vi "指数电流信号.vi"() -> ()   [LabVIEW 2020]
doc: "I. Description:\nThis example demonstrates how to acquire a continuous amount of data (Waveform) using the DAQ device's internal clock.\n\nII. Instructions for Running:\n1. Select the physical channel to correspond to where your signal is input on the DAQ device.\n2. Enter the minimum and maximum voltages.\nNote: For better accuracy try to match the input range to the expected voltage level of the measured signal.\n3. Select the number of samples to acquire per loop iteration.\n4. Set the rate of the acquisition\nNote: The rate should be AT LEAST twice as fast as the maximum frequency component of the signal being acquired.\n\nIII. Block Diagram Steps:\n1. Create an analog input voltage channel.\n2. Set the rate for the sample clock. Additionally, define the sample mode to be continuous.\n3. Call the Start VI to start the acquisition.\n4. Read the waveform data in a loop until the user hits the stop button or an error occurs.\nNote: This example reads data from one or more channels and returns an array of data. Use the Index Array function to access an individual channel of data.\n5. Call the Clear Task VI to clear the Task.\n6. Use the popup dialog box to display an error if any.\n\nIV. I/O Connections Overview:\nMake sure your signal input terminal matches the Physical Channel I/O Control. For further connection information, refer to your hardware reference manual."
uses:
  GlobalVariable.vi
  <vilib>/Analysis/polynomials.llb/Scalar Polynomial Evaluation (DBL).vi
  <vilib>/Analysis/NI_AALPro.lvlib
panel:
  out "实际步长(mS)":u32
  in  "定值电流观测":bool
  in  "二倍周期(秒)":dbl=80.0
  in  "开始自检":bool
  in  "初始I(0)电流(A)":dbl=1e-09
  in  "停止":bool
  in  "当前电流值（A)":dbl format="%#_6e"
  out "偏压(V)":dbl
  out "VI量程":bool[](array[boolean])
  in  "Loop Time (ms)":u32=200 caption="点间隔步长(mS)"
  out "XY Graph":cluster{"Y":dbl[], "Y":dbl[]}[](graph) caption="指数电流输出"
  # "I(t)=I(0)exp(t/Te)"
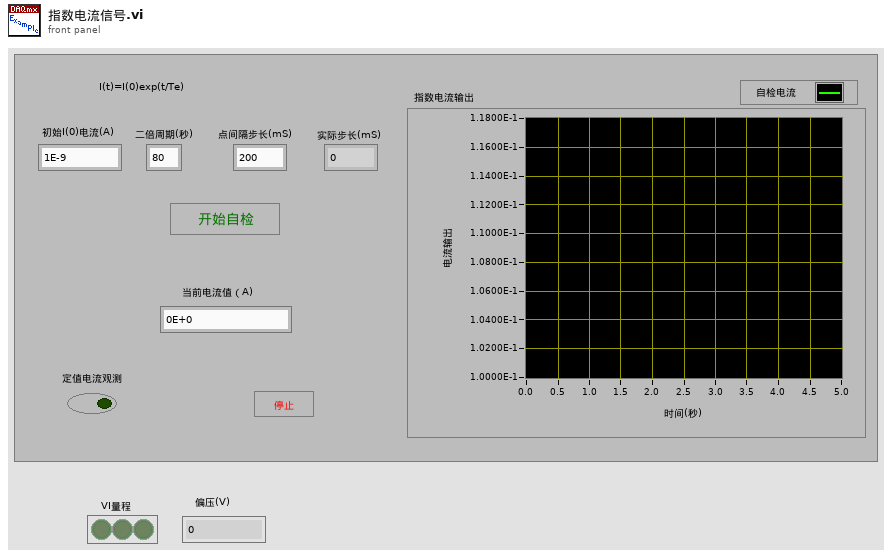
[diagram p1: front panel]
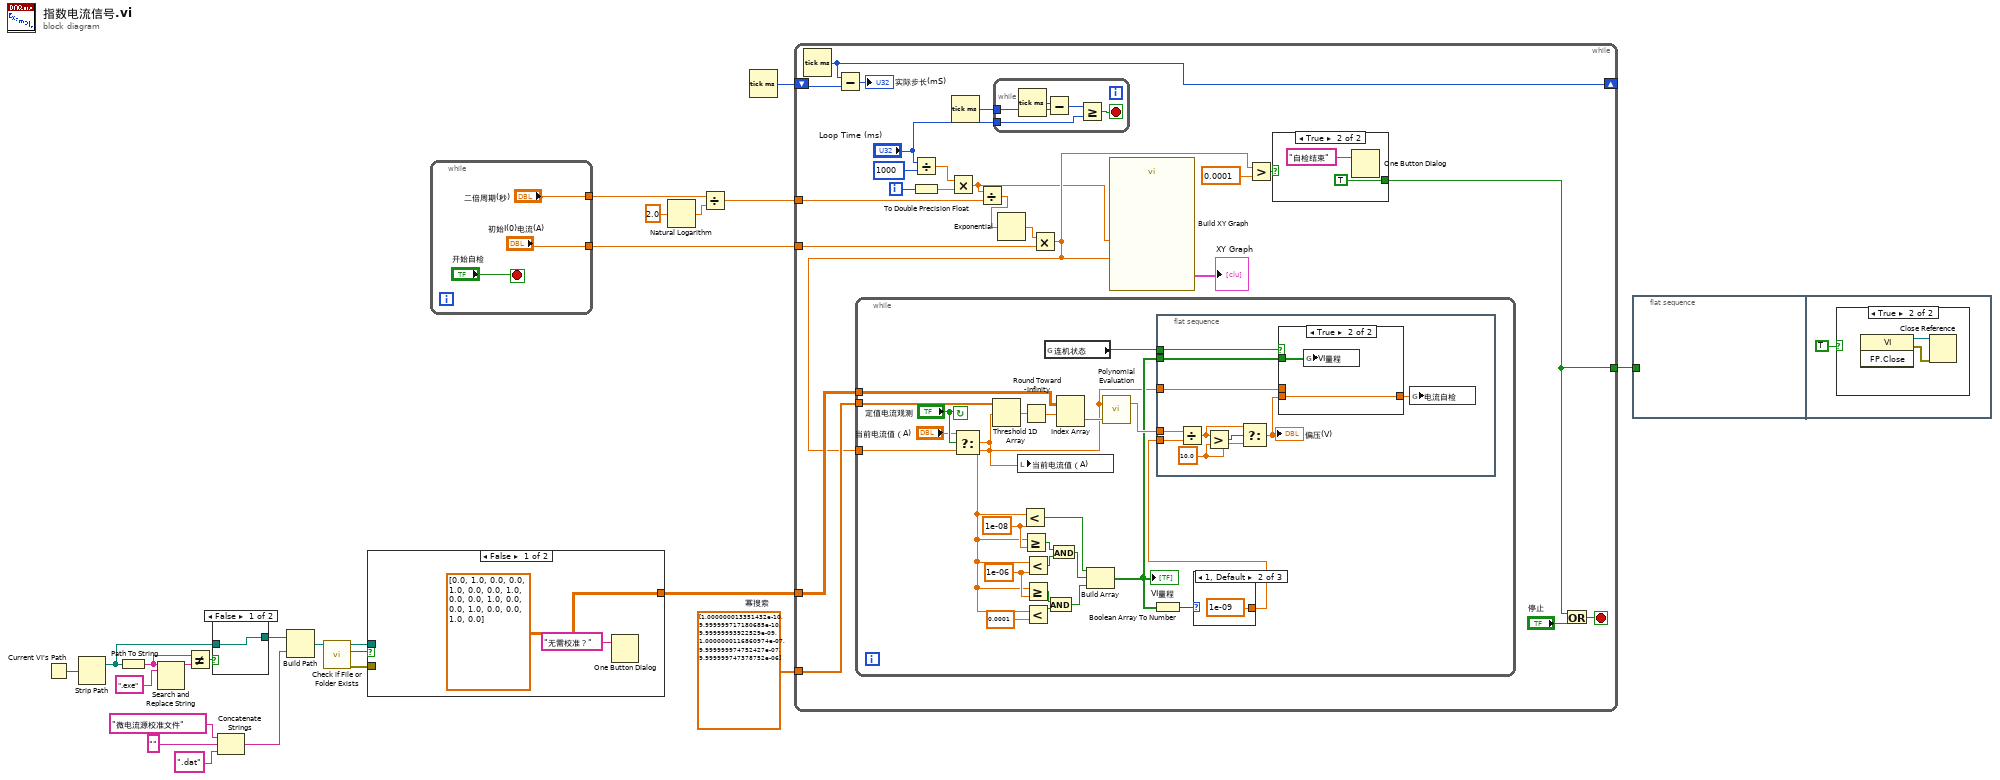
[diagram p0: block diagram]
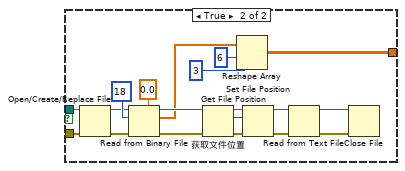
[diagram p2: hidden frame]
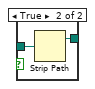
[diagram p4: hidden frame]
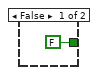
[diagram p5: hidden frame]
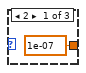
[diagram p7: hidden frame]
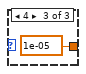
[diagram p8: hidden frame]
diagram:
  w20 = sgl[] [1e-10, 1e-09, 1e-08, 1e-07, 1e-06, 1e-05]  # 幂搜索
  n1 = Current VI's Path() -> (path=w19:path)
  n2 = Strip Path(path=w19) -> (stripped path=w14:path)  [unwired: 1 out]
  n3 = Path To String(path=w14) -> (string=w16:string)
  n4 = Search and Replace String(input string=w16, search string=".exe" ("搜索字符串")) -> (result string=w17:string)  [unwired: 6 in, 3 out]
  n5 = Not Equal?(x=w16, y=w17) -> (x != y?=w15:bool)
  n6 = case shown="False" w15 {
    tunnel: w14 -> [w25 w27]
    tunnel: [w25 w26] -> w13
    frame False {
    }
    frame True {
      n7 = Strip Path(path=w27) -> (stripped path=w26:path)  [unwired: 1 out]
    }
  }
  n8 = Concatenate Strings("微电流源校准文件", "" ("字符串"), ".dat") -> (w8:string)
  n9 = Build Path(base path=w13, name or relative path=w8) -> (appended path=w7:path)
  n10 = call <vilib>:"Check if File or Folder Exists.vi"("path"=w7) -> ("error out"=w4:errorcluster, "file or folder exists?"=w5:bool, "dup path"=w6:path)  [unwired: 8 in]
  n11 = case shown="False" w5 {
    tunnel: [sgl[][] [[0.0, 1.0, 0.0], [0.0, 1.0, 0.0], [0.0, 1.0, 0.0], [0.0, 1.0, 0.0], [0.0, 1.0, 0.0], [0.0, 1.0, 0.0]] w32] -> w12
    tunnel: w6 -> [_ w31]
    tunnel: w4 -> [_ w30]
    frame False {
      n12 = One Button Dialog(message="无需校准？" ("消息")) -> ()  [unwired: 1 in, 1 out]
    }
    frame True {
      n13 = Open/Create/Replace File(file path (use dialog)=w31, error in=w30) -> (refnum out=w37:refnum<file>, error out=w36:errorcluster)  [unwired: 4 in, 1 out]
      n14 = Read from Binary File(5:sgl 0.0 ("byte stream type"), 8:w36, 10:18 ("count"), 11:w37) -> (0:w39:errorcluster, 2:w35:sgl[], 3:w38:refnum<file>)  [unwired: 2 in, 1 out]
      n15 = Get File Position "获取文件位置"(4:w39, 7:w38) -> (0:w47:errorcluster, 2:w46:i64, 3:w48:refnum<file>)
      n16 = Reshape Array(w35, 6 ("维数大小"), 3 ("维数大小")) -> (w32:sgl[][])
      n17 = Set File Position(offset (in bytes) (0)=w46, refnum=w48, error in=w47) -> (refnum out=w45:refnum<file>, error out=w44:errorcluster)  [unwired: 1 in]
      n18 = Read from Text File(file (use dialog)=w45, error in=w44) -> (refnum out=w43:refnum<file>, error out=w42:errorcluster)  [unwired: 1 in, 3 out]
      n19 = Close File(refnum=w43, error in=w42) -> ()  [unwired: 2 out]
    }
  }
  n20 = while {
    tunnel: ["二倍周期(秒)"] -> w22
    tunnel: ["初始I(0)电流(A)"] -> w3
    stop <- "开始自检" stop-if-true
  }
  n21 = Natural Logarithm(1:2.0 ("x")) -> (0:w24:dbl)
  n22 = Divide(x=w22, y=w24) -> (x/y=w21:dbl)
  n23 = Tick Count (ms)() -> (millisecond timer value=w11:u32)
  n24 = while {
    tunnel: w21 -> [w66]
    tunnel: w3 -> [w65]
    tunnel: w12 -> [w63]
    tunnel: w20 -> [w62]
    shift-right: [w54] -> _
    shift-left: w11 -> [w58]
    tunnel: [w52] -> w1
    i -> [w64]
    stop <- w74 stop-if-true
    n25 = Tick Count (ms)() -> (millisecond timer value=w54:u32)
    n26 = Subtract(x=w54, y=w58) -> (x-y=→"实际步长(mS)":u32)
    n27 = Divide(x="Loop Time (ms)", y=u32 1000) -> (x/y=w68:dbl)
    n28 = To Double Precision Float(number=w64) -> (double precision float=w72:dbl)
    n29 = Multiply(x=w68, y=w72) -> (x*y=w55:dbl)
    n30 = Tick Count (ms)() -> (millisecond timer value=w56:u32)
    n31 = Divide(x=w55, y=w66) -> (x/y=w71:dbl)
    n32 = while {
      tunnel: w56 -> [w78]
      tunnel: "Loop Time (ms)" -> [w75]
      stop <- w76 stop-if-true
      n33 = Tick Count (ms)() -> (millisecond timer value=w79:u32)
      n34 = Subtract(x=w79, y=w78) -> (x-y=w77:u32)
      n35 = Greater Or Equal?(x=w77, y=w75) -> (x >= y?=w76:bool)
    }
    n36 = Exponential(1:w71) -> (0:w70:dbl)
    n37 = Multiply(x=w70, y=w65) -> (x*y=w61:dbl)
    n38 = while {
      tunnel: w61 -> [w93]
      tunnel: w63 -> [w89]
      tunnel: w62 -> [w91]
      stop <- "定值电流观测" continue-if-true
      w102 = 1e-06 ("y")
      w105 = 1e-08 ("y")
      n39 = Select(t="当前电流值（A)", s="定值电流观测", f=w93) -> (s? t:f=w84:dbl)
      n40 = Threshold 1D Array(2:w84, 3:w91) -> (0:w90:sgl)  [unwired: 1 in]
      n41 = local write "当前电流值（A)"(w84) -> ()
      n42 = Less?(x=w84, y=w105) -> (x < y?=w98:bool)
      n43 = Round Toward -Infinity(1:w90) -> (0:w88:sgl)
      n44 = Greater Or Equal?(x=w84, y=w105) -> (x >= y?=w103:bool)
      n45 = Less?(x=w84, y=w102) -> (x < y?=w104:bool)
      n46 = Greater Or Equal?(x=w84, y=w102) -> (x >= y?=w101:bool)
      n47 = Less?(x=w84, y=0.0001) -> (x < y?=w100:bool)
      n48 = global read "GlobalVariable.vi" "连机状态"() -> (w83:bool)
      n49 = And(x=w101, y=w100) -> (x .and. y?=w96:bool)
      n50 = And(x=w103, y=w104) -> (x .and. y?=w97:bool)
      n51 = Index Array(array=w89, index (row)=w88) -> (element=w87:sgl[])  [unwired: 1 in]
      n52 = Build Array(w98, w97, w96) -> (w85:bool[])
      "VI量程" <- w85
      n53 = call-poly <vilib>:"Polynomial Evaluation.vi"("P(x)"=w87, "a"=w84) -> ("P(a)"=w86:dbl)  [unwired: 1 out]
      n54 = Boolean Array To Number(Boolean array=w85) -> (number=w106:u32)
      n55 = flat-sequence {
        tunnel: w95 -> [w116]
        tunnel: w85 -> [w115]
        tunnel: w86 -> [w114]
        tunnel: w84 -> [w107]
        tunnel: w83 -> [w109]
        frame #0 {
          w111 = 10.0 ("y")
          n56 = Divide(x=w114, y=w116) -> (x/y=w112:dbl)
          n57 = Greater?(x=w112, y=w111) -> (0:w113:bool)
          n58 = Select(t=w112, s=w113, f=w111) -> (s? t:f=w110:dbl)
          "偏压(V)" <- w110
          n59 = case shown="True" w109 {
            tunnel: w115 -> [_ w119]
            tunnel: w110 -> [_ w118]
            tunnel: [w117 w118] -> w108
            tunnel: w107 -> [w117 _]
            frame False {
            }
            frame True {
              n60 = global write "GlobalVariable.vi" "VI量程"(w119) -> ()
            }
          }
          n61 = global write "GlobalVariable.vi" "电流自检"(w108) -> ()
        }
      }
      n62 = case shown="1, Default" w106 {
        tunnel: [1e-07 ("timeout") 1e-09 ("timeout") 1e-05 ("timeout")] -> w95
        frame 2 {
        }
        frame 1, Default {
        }
        frame 4 {
        }
      }
    }
    n63 = call "Build XY Graph"("Y Input"=w61, "X Input"=w55) -> ("XY Graph"=→"XY Graph":cluster{"Y":dbl[], "Y":dbl[]}[])  [unwired: 3 in, 6 out]
    n64 = Greater?(x=w61, y=0.0001) -> (0:w59:bool)
    n65 = case shown="True" w59 {
      tunnel: [FALSE ("x或y?") TRUE ("x或y?")] -> w52
      frame False {
      }
      frame True {
        n66 = One Button Dialog(message="自检结束" ("消息")) -> ()  [unwired: 1 in, 1 out]
      }
    }
    n67 = Or(x=w52, y="停止") -> (x .or. y?=w74:bool)
  }
  n68 = flat-sequence {
    tunnel: w1 -> [_]
    frame #0 {
    }
    frame #1 {
      n69 = case shown="True" TRUE {
        frame False {
        }
        frame True {
          n70 = invoke class="VI" method="FP.Close"() -> (reference out=w125:refnum<vi>, error out=w124:errorcluster)  [unwired: 3 in, 1 out]
          n71 = Close Reference(reference=w125, error in (no error)=w124) -> ()  [unwired: 1 out]
        }
      }
    }
  }
